vi "Get Server Certificate File.vi"(11 "OOP Server in":refnum<class "ctet_dio.lvclass">) -> (2 "Server Certificate File (.crt)":path, 3 "OOP Server out":refnum<class "ctet_dio.lvclass">)   [LabVIEW 2019, in "ctet_dio.lvlib" / "ctet_dio.lvclass"]
uses:
  ctet_dio.lvclass
  ctet_dio.lvclass/ctet_dio.ctl
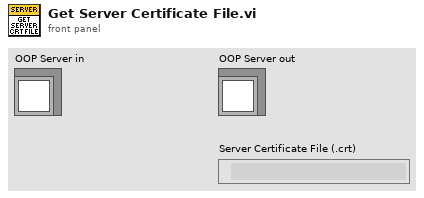
[diagram p1: front panel]
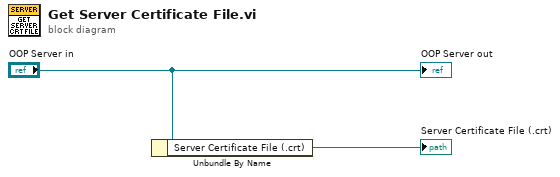
[diagram p0: block diagram]
diagram:
  n1 = Unbundle By Name("OOP Server in") -> ("Server Certificate File (.crt)"=→"Server Certificate File (.crt)":path)
  "OOP Server out" <- "OOP Server in"
